vi "Read Rotation.vi"(8 "error in (no error)":errorcluster, 11 "Gyro Bias":dbl) -> (0 "error out":errorcluster, 3 "Z Rotation (rads)":dbl)   [LabVIEW 2018]
uses:
  <vilib>/Analysis/coordinate.llb/Angle Range (Degree).ctl
  <vilib>/Analysis/coordinate.llb/Angle Units.ctl
  <vilib>/Analysis/coordinate.llb/Wrap Angle (scalar).vi
  Gyro Globals.vi
  lib/MPU6050 Read Rotation Data.vi
  lib/Calculate Orientation.vi
  <vilib>/Analysis/NI_AAL_Angle.lvlib
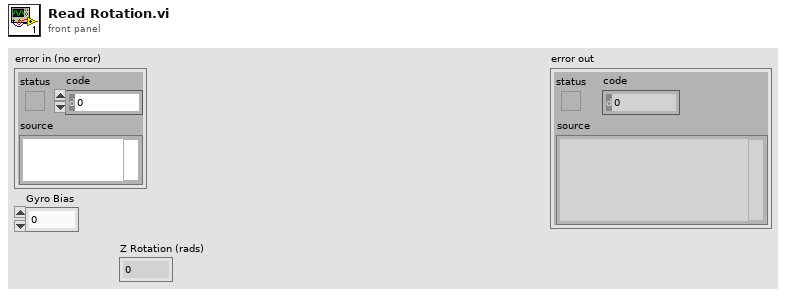
[diagram p1: front panel]
types:
  T1 = typedef "NI_AAL_Angle.lvlib/Angle Units.ctl" = i32
  T2 = typedef "NI_AAL_Angle.lvlib/Angle Range (Degree).ctl" = u16
  T3 = typedef "I2C.lvlib/I2C Reference.ctl" = cluster{"myRIO Reference":T4, "I2C Channels Enum":T8, "I2C Configuration":T9}
  T4 = typedef "myRIO Generic Hardware Reference.ctl" = cluster{"myRIO Model":T5, "myRIO Hardware Reference":T6}
  T5 = typedef "Hardware Version Enum.ctl" = enum16{"Unknown", "myRIO-1900", "myRIO-1950", "roboRIO", "NI ELVIS RIO CM", "ELVIS III"}
  T6 = typedef "myRIO v1.0 Reference.ctl" = cluster{"Generic FPGA Reference":T7, "Allow multiple opens":bool}
  T7 = typedef "Generic FPGA Reference.ctl" = refnum<k20>
  T8 = typedef "I2C Channels Enum.ctl" = enum16{"Not Connected", "A/I2C", "B/I2C", "I2C/I2C"}
  T9 = typedef "I2C.lvlib/I2C Configuration.ctl" = cluster{"I2C Transfer Rate":T10}
  T10 = typedef "I2C.lvlib/I2C Transfer Rate.ctl" = enum16{"Standard mode (100 kbps)", "Fast mode (400 kbps)"}
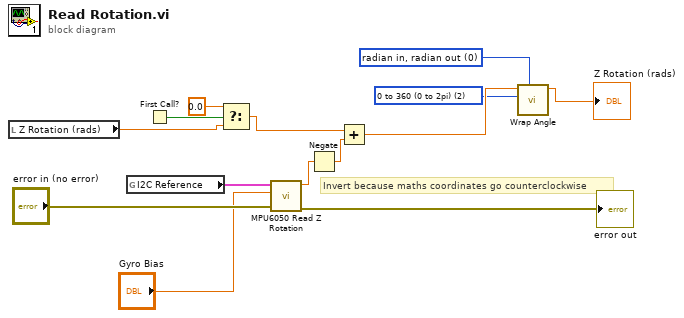
[diagram p0: block diagram]
diagram:
  w5 = T1 0 items=["radian in, radian out", "radian in, degree out", "degree in, degree out", "degree in, radian out"] ("angle units")
  w6 = T2 2 items=["none", "-180 to 180 (-pi to pi)", "0 to 360 (0 to 2pi)"] ("angle range")
  # "Invert because maths coordinates go counterclockwise"
  n1 = local read "Z Rotation (rads)"() -> (w10:dbl)
  n2 = global read "Gyro Globals.vi" "I2C Reference"() -> (w14:T3)
  n3 = First Call?() -> (First Call?: T/F=w11:bool)
  n4 = Select(t=0.0, s=w11, f=w10) -> (s? t:f=w9:dbl)
  n5 = call "MPU6050 Read Z Rotation.vi"("error in (no error)"="error in (no error)", "Gyro Bias"="Gyro Bias", "I2C Ref In"=w14) -> ("error out"=→"error out":errorcluster, "Z Rotation (rads)"=w2:dbl)  [unwired: 7 in]
  n6 = Negate(x=w2) -> (-x=w3:dbl)
  n7 = Add(x=w9, y=w3) -> (x+y=w7:dbl)
  n8 = call-poly <vilib>:"Wrap Angle.vi"("angle units"=w5, "angle range"=w6, "angle in"=w7) -> ("angle out"=→"Z Rotation (rads)":dbl)  [unwired: 7 in, 1 out]
